vi "Wrapper VIs Paths.vi"(8 "error in (no error)":errorcluster, 9 "Op":enum16{"Get", "Add", "Clear"}(ring), 11 "Path":path) -> (0 "error out":errorcluster, 3 "Array":path[](array[path]))   [LabVIEW 2020, in "WebServiceImporter.lvlib" / "VI Generator.lvlib"]
uses:
  <vilib>/Platform/WebService/VI Generator/VI Generator.lvlib
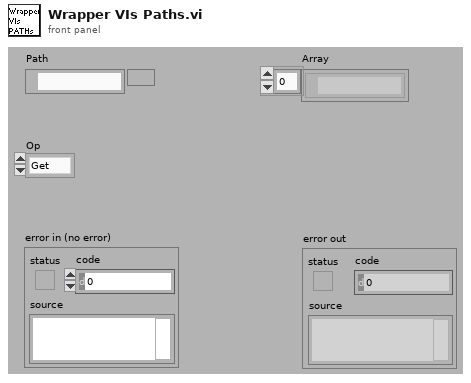
[diagram p1: front panel]
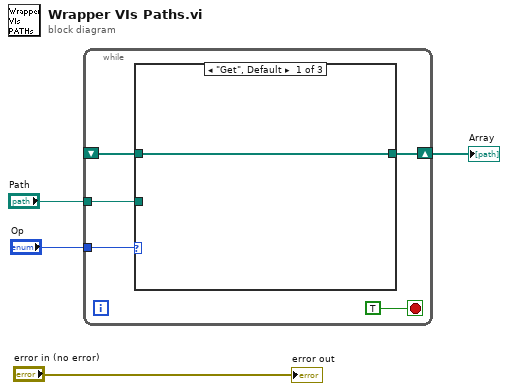
[diagram p0: block diagram]
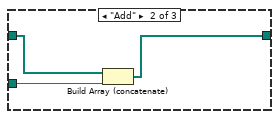
[diagram p2: hidden frame]
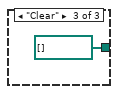
[diagram p3: hidden frame]
diagram:
  n1 = while {
    tunnel: "Op" -> [w8]
    tunnel: "Path" -> [w7]
    shift-right: [w6] -> w1
    shift-left: _ -> [w5]
    stop <- TRUE stop-if-true
    n2 = case shown="\"Get\", Default" w8 {
      tunnel: w7 -> [_ w13 _]
      tunnel: [w10 w12 path[] []] -> w6
      tunnel: w5 -> [w10 w11 _]
      frame "Get", Default {
      }
      frame "Add" {
        n3 = Build Array (concatenate)(w11, w13) -> (w12:path[])
      }
      frame "Clear" {
      }
    }
  }
  "Array" <- w1
  "error out" <- "error in (no error)"
